vi "BPM FPGA.vi"() -> ()   [LabVIEW 2016]
uses:
  <vilib>/Platform/TimedLoop/XDataNode/timing_clust.ctl
  <vilib>/Platform/TimedLoop/XDataNode/nitl_modes.ctl
  <vilib>/Platform/TimedLoop/XDataNode/wakeup.ctl
  <vilib>/rvi/FXPMathLib/basic elements/FxpIntAccumulator/subVIs/nifxpmath_IntAccumulator_SimConfig.ctl
  <vilib>/rvi/Emulation/niFpgaGetClockAttributes.vi
  <vilib>/rvi/Emulation/niFpgaSctlEmulationGetInTimedLoop.vi
  <vilib>/rvi/Emulation/niFpgaEmulationReportErrorSimple.vi
  <vilib>/rvi/eio/common/nirviEmuTemplateMethod_errors.vi
  <vilib>/rvi/Emulation/niFpgaCriticalErrorInLSC.vi
  <vilib>/rvi/Analysis/common/codeGenErrors/XNode/niFpgaXNodeCodeGenErrorHandle.vi
  <vilib>/rvi/FXPMathLib/basic elements/FxpIntAccumulator/simVIs/DllFxpIntAccumulator_sub.vi
  <vilib>/eio/EIONode/EIONode.xnode
  <vilib>/rvi/Analysis/measure/dc-rms/XNode/niFpgaDC-RMS.xnode
  <vilib>/Platform/TimedLoop/XDataNode/XDataNode.xnode
  <vilib>/rvi/FXPMathLib/basic elements/FxpIntAccumulator/XNode/nifxpmath_IntAccumulator.xnode
  <vilib>/rvi/FXPMathLib/FxpMul/XNode/nifxpmath_Multiplier.xnode
  <vilib>/Platform/TimedLoop/XDataNode/XDNodeRunTimeDep.lvlib
  <vilib>/rvi/FXPMathLib/sim/FxpSim.dll
panel:
  in  "einzel readbacks setpoints":fxp<+/-,26,5>[](array[numeric])=[0.0, 0.0, 0.0, 0.0, 0.0, 0.0, 0.0, 0.0, 0.0] format="%.23g"
  out "terminal voltage":fxp<+/-,26,5> format="%.23g"
  out "einzel readbacks readbacks":fxp<+/-,26,5>[](array[numeric]) format="%.23g"
  out "chop output":fxp<+/-,26,5>
  out "Analog input":fxp<+/-,26,5>[](array[numeric]) format="%.23g"
  in  "BPM":bool[](array[boolean])=[FALSE, FALSE, FALSE, FALSE, FALSE, FALSE, FALSE, FALSE]
  # "0 run\n1 divert\n2 offset\n3 chop to detector"
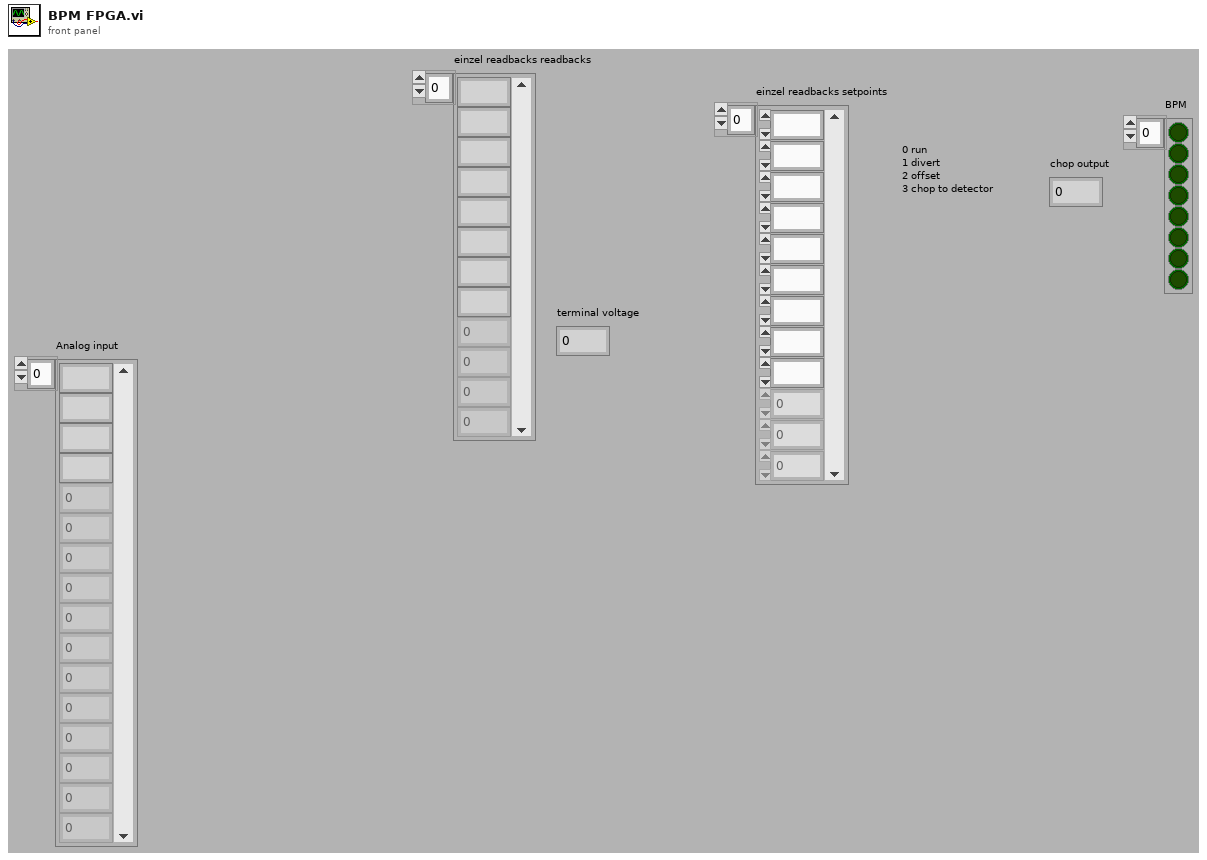
[diagram p1: front panel]
types:
  T1 = typedef "XDNodeRunTimeDep.lvlib/timing_clust.ctl" = cluster{"Expected End [f-1]":u64, "Actual End [f-1]":u64, "Finished Late? [f-1]":bool, "Expected End [i-1]":u64, "Actual End [i-1]":u64, "Finished Late? [i-1]":bool, "Expected Start [i]":u64, "Actual Start [i]":u64, "Expected Start [f]":u64, "Actual Start [f]":u64, "Source Name":string, "Structure Name":string, "Period":i64, "Deadline":i64, "Offset":i64, "Start":i64, "Priority":i32, "Timeout":i32, "Mode":T2, "Wakeup Reason":T3, "Error":errorcluster, "Source Type":string, "Secondary Source Type":string, "Global End Time":u64, "Global Start Time":u64, "Frame Duration":u64, "Iteration Duration":u64, "Assigned CPU":i32, "I/O Scan Engine Mode":u32}
  T2 = typedef "XDNodeRunTimeDep.lvlib/nitl_modes.ctl" = enum32{"No Change", "Process missed periods, maintain original phase", "Discard missed periods, maintain original phase", "Process missed periods, ignore original phase", "Discard missed periods, ignore original phase"}
  T3 = typedef "XDNodeRunTimeDep.lvlib/wakeup.ctl" = enum32{"Normal", "Aborted", "Asynchronous wakeup", "Timing source error", "Timed loop error", "Timeout"}
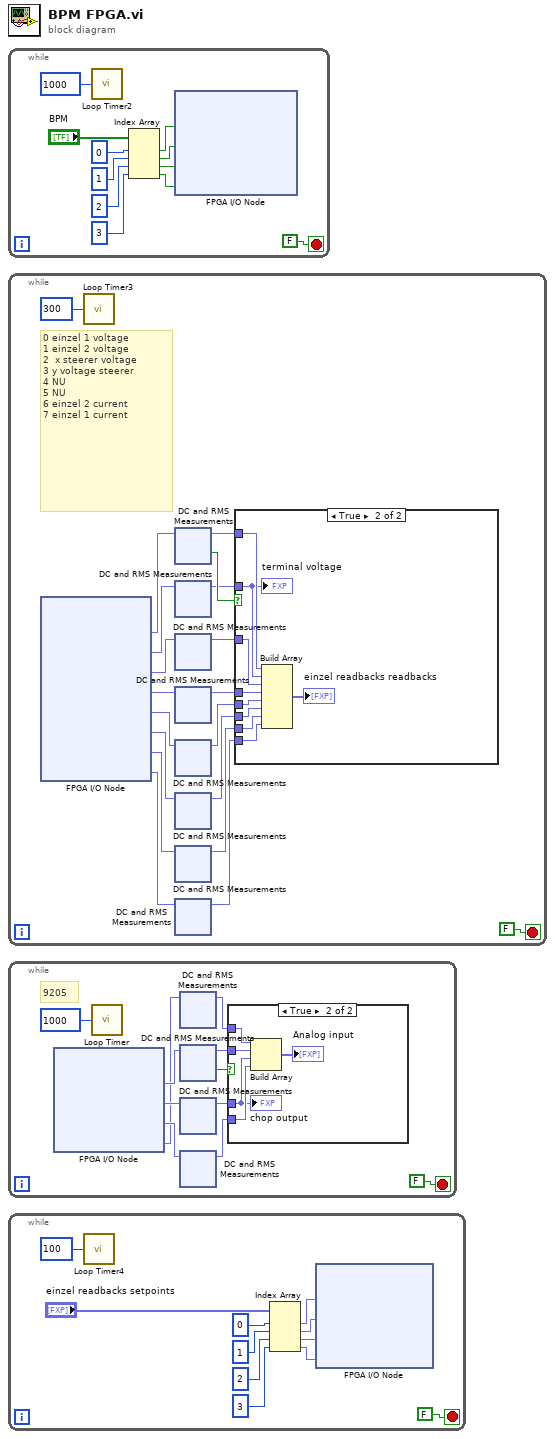
[diagram p0: block diagram]
diagram:
  n1 = while {
    stop <- FALSE stop-if-true
    n2 = call "Loop Timer2"("Count(mSec)"=u32 1000 ("Count(Ticks)")) -> ()  [unwired: 1 out]
    n3 = Index Array(array="BPM", index #1=0 ("index"), index #2=1 ("index"), index #3=2 ("index"), index #4=3 ("index")) -> (element #1=w1:bool, element #2=w7:bool, element #3=w8:bool, element #4=w9:bool)
    n4 = xnode "FPGA I/O Node"("Mod1/DIO0"=w1, "Mod1/DIO1"=w7, "Mod1/DIO2"=w8, "Mod1/DIO3"=w9) -> ()  [unwired: 4 in, 4 out]
  }
  n5 = while {
    stop <- FALSE stop-if-true
    # "0 einzel 1 voltage\n1 einzel 2 voltage\n2  x steerer voltage\n3 y voltage steerer\n4 NU\n5 NU\n6 einzel 2 current\n7 einzel 1 current"
    n6 = xnode "FPGA I/O Node"() -> ("Mod4/AI0"=w28:fxp<+/-,16,5>, "Mod4/AI1"=w25:fxp<+/-,16,5>, "Mod4/AI2"=w24:fxp<+/-,16,5>, "Mod4/AI3"=w23:fxp<+/-,16,5>, "Mod4/AI4"=w22:fxp<+/-,16,5>, "Mod4/AI5"=w17:fxp<+/-,16,5>, "Mod4/AI6"=w15:fxp<+/-,16,5>, "Mod4/AI7"=w13:fxp<+/-,16,5>)  [unwired: 8 in, 8 out]
    n7 = call "Loop Timer3"("Count(uSec)"=u32 300 ("Count(Ticks)")) -> ()  [unwired: 1 out]
    n8 = xnode "DC and RMS Measurements"("input data"=w28) -> ("DC"=w26:fxp<+/-,16,5>, "output valid"=w27:bool)  [unwired: 1 in]
    n9 = xnode "DC and RMS Measurements"("input data"=w25) -> ("DC"=w21:fxp<+/-,16,5>)  [unwired: 1 in, 1 out]
    n10 = xnode "DC and RMS Measurements"("input data"=w24) -> ("DC"=w20:fxp<+/-,16,5>)  [unwired: 1 in, 1 out]
    n11 = xnode "DC and RMS Measurements"("input data"=w23) -> ("DC"=w19:fxp<+/-,16,5>)  [unwired: 1 in, 1 out]
    n12 = xnode "DC and RMS Measurements"("input data"=w22) -> ("DC"=w18:fxp<+/-,16,5>)  [unwired: 1 in, 1 out]
    n13 = xnode "DC and RMS Measurements"("input data"=w17) -> ("DC"=w16:fxp<+/-,16,5>)  [unwired: 1 in, 1 out]
    n14 = xnode "DC and RMS Measurements"("input data"=w15) -> ("DC"=w14:fxp<+/-,16,5>)  [unwired: 1 in, 1 out]
    n15 = xnode "DC and RMS Measurements"("input data"=w13) -> ("DC"=w12:fxp<+/-,16,5>)  [unwired: 1 in, 1 out]
    n16 = case shown="True" w27 {
      tunnel: w26 -> [_ w678]
      tunnel: w21 -> [_ w671]
      tunnel: w20 -> [_ w677]
      tunnel: w19 -> [_ w676]
      tunnel: w18 -> [_ w675]
      tunnel: w16 -> [_ w674]
      tunnel: w14 -> [_ w673]
      tunnel: w12 -> [_ w672]
      frame False {
      }
      frame True {
        n17 = Build Array(w678, w671, w677, w676, w675, w674, w673, w672) -> (→"einzel readbacks readbacks":fxp<+/-,16,5>[])
        "terminal voltage" <- w671
      }
    }
  }
  n18 = while {
    stop <- FALSE stop-if-true
    # "9205"
    n19 = xnode "FPGA I/O Node"() -> ("Mod3/AI0"=w686:fxp<+/-,26,5>, "Mod3/AI1"=w685:fxp<+/-,26,5>, "Mod3/AI2"=w684:fxp<+/-,26,5>, "Mod3/AI3"=w683:fxp<+/-,26,5>)  [unwired: 4 in, 4 out]
    n20 = call "Loop Timer"("Count(Ticks)"=u32 1000) -> ()  [unwired: 1 out]
    n21 = xnode "DC and RMS Measurements"("input data"=w683) -> ("DC"=w682:fxp<+/-,26,5>)  [unwired: 1 in, 1 out]
    n22 = xnode "DC and RMS Measurements"("input data"=w686) -> ("DC"=w687:fxp<+/-,26,5>, "output valid"=w688:bool)  [unwired: 1 in]
    n23 = xnode "DC and RMS Measurements"("input data"=w685) -> ("DC"=w680:fxp<+/-,26,5>)  [unwired: 1 in, 1 out]
    n24 = xnode "DC and RMS Measurements"("input data"=w684) -> ("DC"=w681:fxp<+/-,26,5>)  [unwired: 1 in, 1 out]
    n25 = case shown="True" w688 {
      tunnel: w687 -> [_ w933]
      tunnel: w682 -> [_ w935]
      tunnel: w681 -> [_ w934]
      tunnel: w680 -> [_ w932]
      frame False {
      }
      frame True {
        n26 = Build Array(w935, w933, w932, w934) -> (→"Analog input":fxp<+/-,26,5>[])
        "chop output" <- w932
      }
    }
  }
  n27 = while {
    stop <- FALSE stop-if-true
    n28 = call "Loop Timer4"("Count(mSec)"=u32 100 ("Count(Ticks)")) -> ()  [unwired: 1 out]
    n29 = Index Array(array="einzel readbacks setpoints", index #1=0 ("index"), index #2=1 ("index"), index #3=2 ("index"), index #4=3 ("index")) -> (element #1=w1020:fxp<+/-,26,5>, element #2=w1019:fxp<+/-,26,5>, element #3=w1018:fxp<+/-,26,5>, element #4=w1017:fxp<+/-,26,5>)
    n30 = xnode "FPGA I/O Node"("Mod2/AO0"=w1020, "Mod2/AO1"=w1019, "Mod2/AO2"=w1018, "Mod2/AO3"=w1017) -> ()  [unwired: 4 in, 4 out]
  }
